vi "get Pmu Real Data.vi"(7 "pmuIndex":i32, 9 "pseudoPdcId":i32, 10 "status":cluster{}, 11 "rd":T1) -> (1 "function return":i32, 2 "status out":cluster{}, 3 "rd out":T1)   [LabVIEW 2012, in "C37118-DLL.lvlib" / "StrongridDLL.lvlib"]
doc: "STRONGRIDIEEEC37118DLL_API int __cdecl getPmuRealData(pmuDataFrame* rd, PmuStatus* status, int32_t pseudoPdcId, int32_t pmuIndex);"
uses:
  StrongridDLL.lvlib
  StrongridDLL.dll
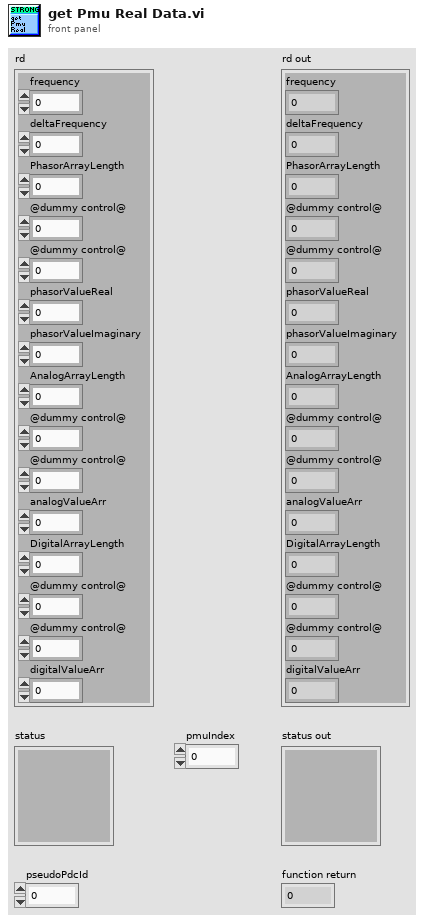
[diagram p1: front panel]
types:
  T1 = cluster{"frequency":sgl, "deltaFrequency":sgl, "PhasorArrayLength":u16, "@dummy control@":i8, "@dummy control@":i8, "phasorValueReal":u32, "phasorValueImaginary":u32, "AnalogArrayLength":u16, "@dummy control@":i8, "@dummy control@":i8, "analogValueArr":u32, "DigitalArrayLength":u16, "@dummy control@":i8, "@dummy control@":i8, "digitalValueArr":u32}
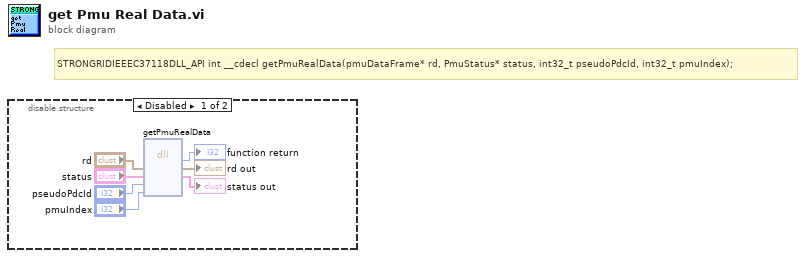
[diagram p0: block diagram]
diagram:
  # "STRONGRIDIEEEC37118DLL_API int __cdecl getPmuRealData(pmuDataFrame* rd, PmuStatus* status, int32_t pseudoPdcId, int32_t pmuIndex);"
  n1 = disable-structure shown="Disabled" {
    frame Disabled {
      n2 = dll-call lib="C:/__TSD-SVN/AFS171 Statnett License PMU Reference Library/source/LabVIEW PRL Library/c37118-dll/labview/vi/Auto Generated/StrongridDLL.*" fn="getPmuRealData"("rd"="rd", "status"="status", "pseudoPdcId"="pseudoPdcId", "pmuIndex"="pmuIndex") -> (→"function return":i32, "rd"=→"rd out":T1, "status"=→"status out":cluster{})  [unwired: 5 in, 2 out]
    }
    frame Enabled {
    }
  }
